vi "Write DMM Setting.vi"(8 "error in (no error)":errorcluster, 10 "DMM Setting":T1={"Function"="DC Volts", "CurrentSource"="1mA", "Resolution"="5 1/2", "Range"=0.5} {"Range" format="%#_f"}, 11 "DMM configuration in":refnum<class "DMM configuration.lvclass">) -> (0 "error out":errorcluster, 3 "DMM configuration out":refnum<class "DMM configuration.lvclass">)   [LabVIEW 2025, in "DMM.lvlib" / "DMM configuration.lvclass"]
uses:
  DMM configuration.lvclass
  DMM Setting.ctl
  DMM configuration.lvclass/DMM configuration.ctl
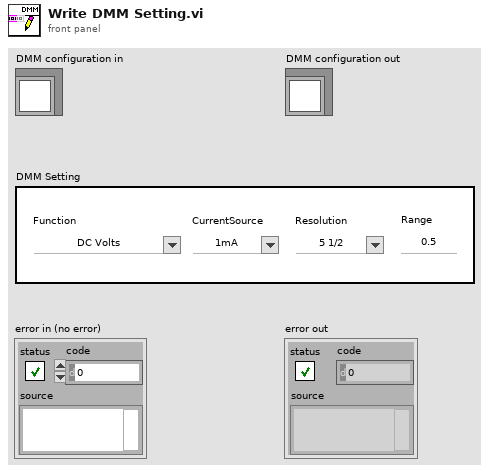
[diagram p1: front panel]
types:
  T1 = typedef "DMM.lvlib/DMM configuration.lvclass/DMM Setting.ctl" = cluster{"Function":string, "CurrentSource":string, "Resolution":string, "Range":dbl}
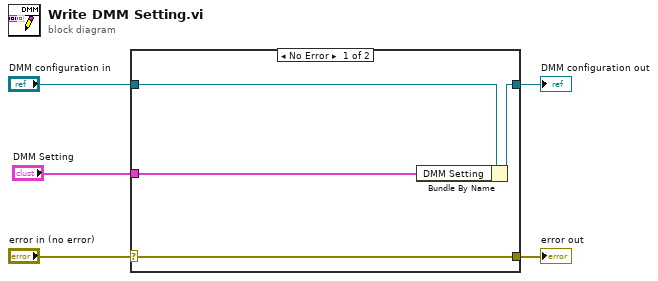
[diagram p0: block diagram]
diagram:
  n1 = case shown="No Error" "error in (no error)" {
    selector: "error in (no error)" -> [w9 w10]
    tunnel: [w9 w10] -> w4
    tunnel: [w7 w11] -> w2
    tunnel: "DMM configuration in" -> [w8 w11]
    tunnel: "DMM Setting" -> [w6 _]
    frame No Error {
      n2 = Bundle By Name(cluster=w8, "DMM Setting"=w6) -> (w7:refnum<class "DMM configuration.lvclass">)
    }
    frame Error {
    }
  }
  "error out" <- w4
  "DMM configuration out" <- w2
